vi "ConvertErdsVersion.vi"(7 "Erds_Version":cluster{"ERD Number":u16, "Data":string}[](array[cluster]), 11 "error in":errorcluster) -> (8 "Version out":T1, 15 "error out":errorcluster)   [LabVIEW 2021]
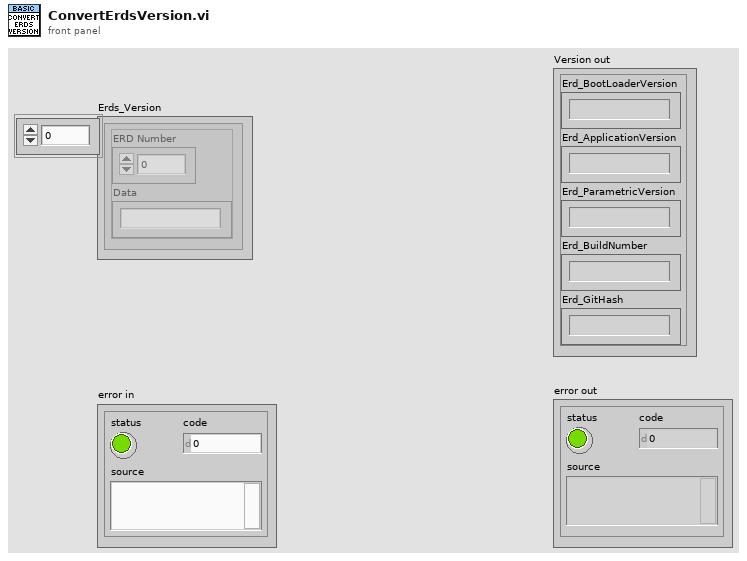
[diagram p1: front panel]
types:
  T1 = cluster{"Erd_BootLoaderVersion":string, "Erd_ApplicationVersion":string, "Erd_ParametricVersion":string, "Erd_BuildNumber":string, "Erd_GitHash":string}
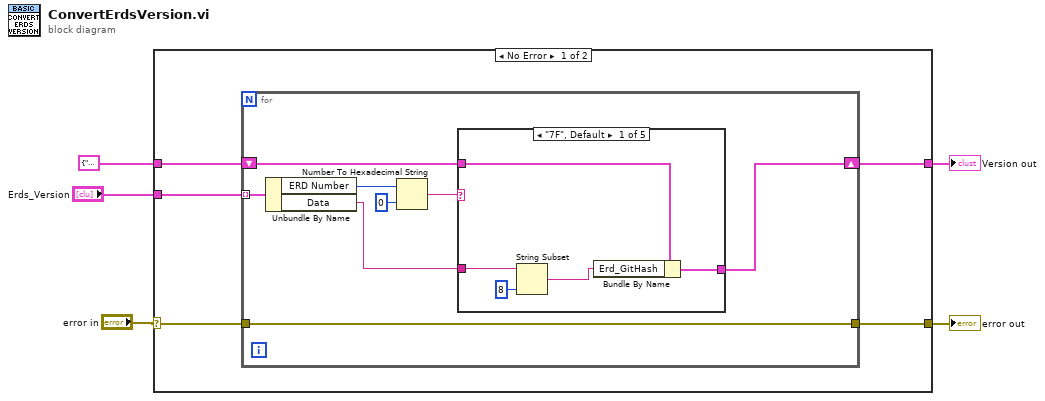
[diagram p0: block diagram]
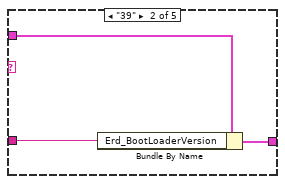
[diagram p2: hidden frame]
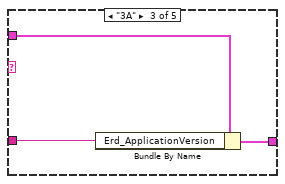
[diagram p3: hidden frame]
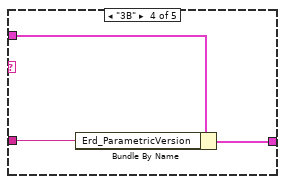
[diagram p4: hidden frame]
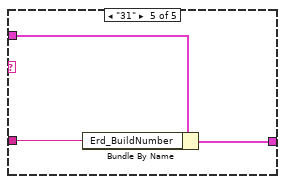
[diagram p5: hidden frame]
diagram:
  n1 = case shown="No Error" "error in" {
    selector: "error in" -> [w8 w36]
    tunnel: "Erds_Version" -> [w10 _]
    tunnel: [w9 w37] -> w4
    tunnel: [w7 w36] -> w1
    tunnel: T1 {"Erd_BootLoaderVersion"="", "Erd_ApplicationVersion"="", "Erd_ParametricVersion"="", "Erd_BuildNumber"="", "Erd_GitHash"=""} ("Version in") -> [w6 w37]
    frame No Error {
      n2 = for {
        tunnel: w10 -> [w18] mode=indexing
        shift-right: [w14] -> w9
        shift-left: w6 -> [w13]
        tunnel: w8 -> [w11]
        tunnel: [w11] -> w7
        n3 = Unbundle By Name(w18) -> ("ERD Number"=w17:u16, "Data"=w15:string)
        n4 = Number To Hexadecimal String(1:i16 0 ("width (-)"), 2:w17) -> (0:w16:string)
        n5 = case shown="\"7F\", Default" w16 {
          tunnel: w15 -> [w21 w26 w29 w32 w35]
          tunnel: [w23 w25 w28 w31 w34] -> w14
          tunnel: w13 -> [w19 w24 w27 w30 w33]
          frame "7F", Default {
            n6 = String Subset(string=w21, length (rest)=8 ("length (rest)")) -> (substring=w20:string)  [unwired: 1 in]
            n7 = Bundle By Name(cluster=w19, "Erd_GitHash"=w20) -> (w23:T1)
          }
          frame "39" {
            n8 = Bundle By Name(cluster=w24, "Erd_BootLoaderVersion"=w26) -> (w25:T1)
          }
          frame "3A" {
            n9 = Bundle By Name(cluster=w27, "Erd_ApplicationVersion"=w29) -> (w28:T1)
          }
          frame "3B" {
            n10 = Bundle By Name(cluster=w30, "Erd_ParametricVersion"=w32) -> (w31:T1)
          }
          frame "31" {
            n11 = Bundle By Name(cluster=w33, "Erd_BuildNumber"=w35) -> (w34:T1)
          }
        }
      }
    }
    frame Error {
    }
  }
  "Version out" <- w4
  "error out" <- w1
